vi "ExampleClient.vi"() -> ()   [LabVIEW 2017]
uses:
  Support/StreamClientState.ctl
  Controller/Support/StreamHeader.ctl
  jsonRPCwebservice/client/config.ctl
  Support/msg.ctl
  <userlib>/_SEH/Controls/CEH/CEH Actions.ctl
  Controller/Support/methods.ctl
  Support/globals.vi
  <vilib>/LVH/i3 JSON/JSON Parsing/Get Object Parameter Files/Get Object Parameter - Object.vi
  <vilib>/WebDAVClient/Simple Get File.vi
  jsonRPCwebservice/client/JSON_RPC_client.lvlib
  <vilib>/LVH/i3 JSON/i3-json.lvlib
  <vilib>/WebDAVClient/NI_WebDAV.lvlib
panel:
  in  "Trace":string
  in  "Tab Control":enum32{"Commands", "Stream", "Files"}(tab)
  in  "ToEcho":string
  in  "CheckConnection":bool
  in  "GoToSafeState":bool
  in  "GetResourceUsage":bool
  in  "echo":bool
  out "logging":bool
  out "Waveforms":sgl[][](graph)
  in  "Stream":bool
  in  "StreamAndLog":bool
  in  "StopStreaming":bool
  in  "ForceTigger":bool
  in  "RefreshLogFiles":bool
  in  "Logs":i32(listbox)
  in  "Download":bool
  in  "Exit":bool
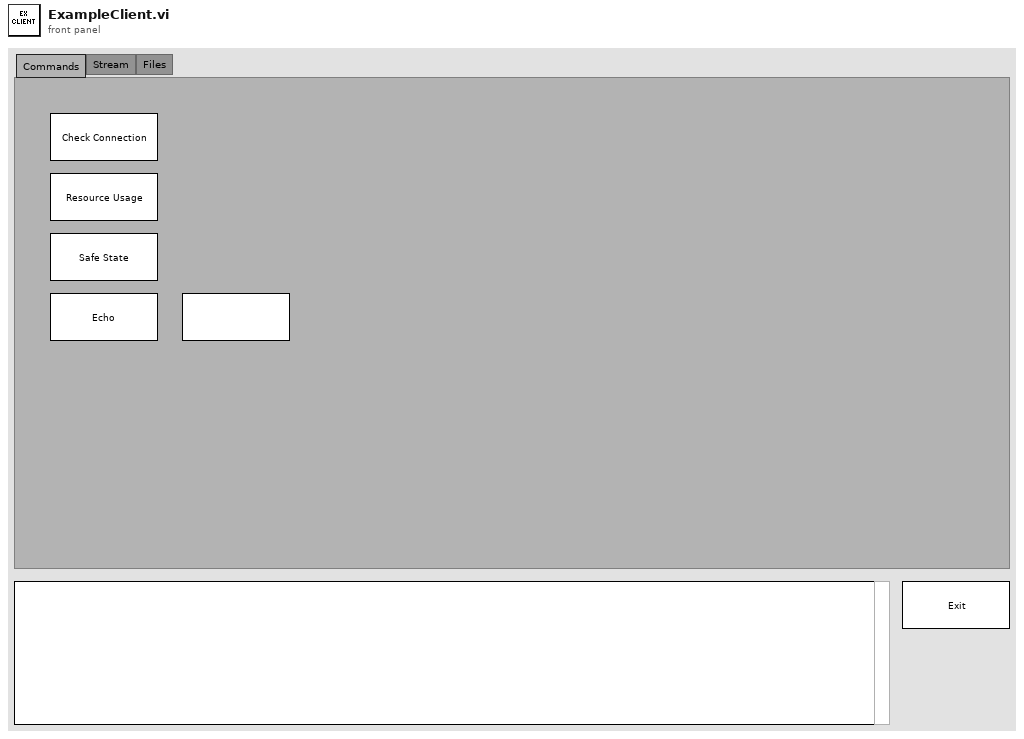
[diagram p1: front panel]
types:
  T1 = typedef "msg.ctl" = cluster{"cmd":string, "parameters":variant}
  T2 = typedef "JSON_RPC_client.lvlib/config.ctl" = cluster{"ip":string, "port":i32, "username":string, "password":string}
  T3 = typedef "StreamHeader.ctl" = cluster{"Channels":string[], "SampleRate":i32}
  T4 = typedef "StreamClientState.ctl" = enum16{"Initialize", "Idle", "ConnectAndOpen", "Connecting", "ReadHeader", "Streaming", "Disconnecting"}
  T5 = enum8{"Enabled", "Disabled", "Disabled and Grayed Out"}
  T6 = typedef "JSON_RPC_client.lvlib/reference.ctl" = cluster{"client handle":T7, "url":string}
  T7 = typedef "LabVIEWHTTPClient.lvlib/ClientHandle.ctl" = refnum<k1>
  T8 = enum16{"open", "open or create", "create or replace", "create", "open (read-only)"}
  T9 = typedef "methods.ctl" = enum16{"none", "echo", "GetResourceUsage", "CheckConnection", "GoToSafeState", "AvailableLogs", "ForceLogTrigger"}
  T10 = typedef "SEH Notification Info.ctl" = cluster{"Priority":i32, "Occurrences":i32, "First Occurrence":timestamp}
  T11 = typedef "CEH Actions.ctl" = enum16{"Log", "Display Error Message", "Safe State", "Shutdown"}
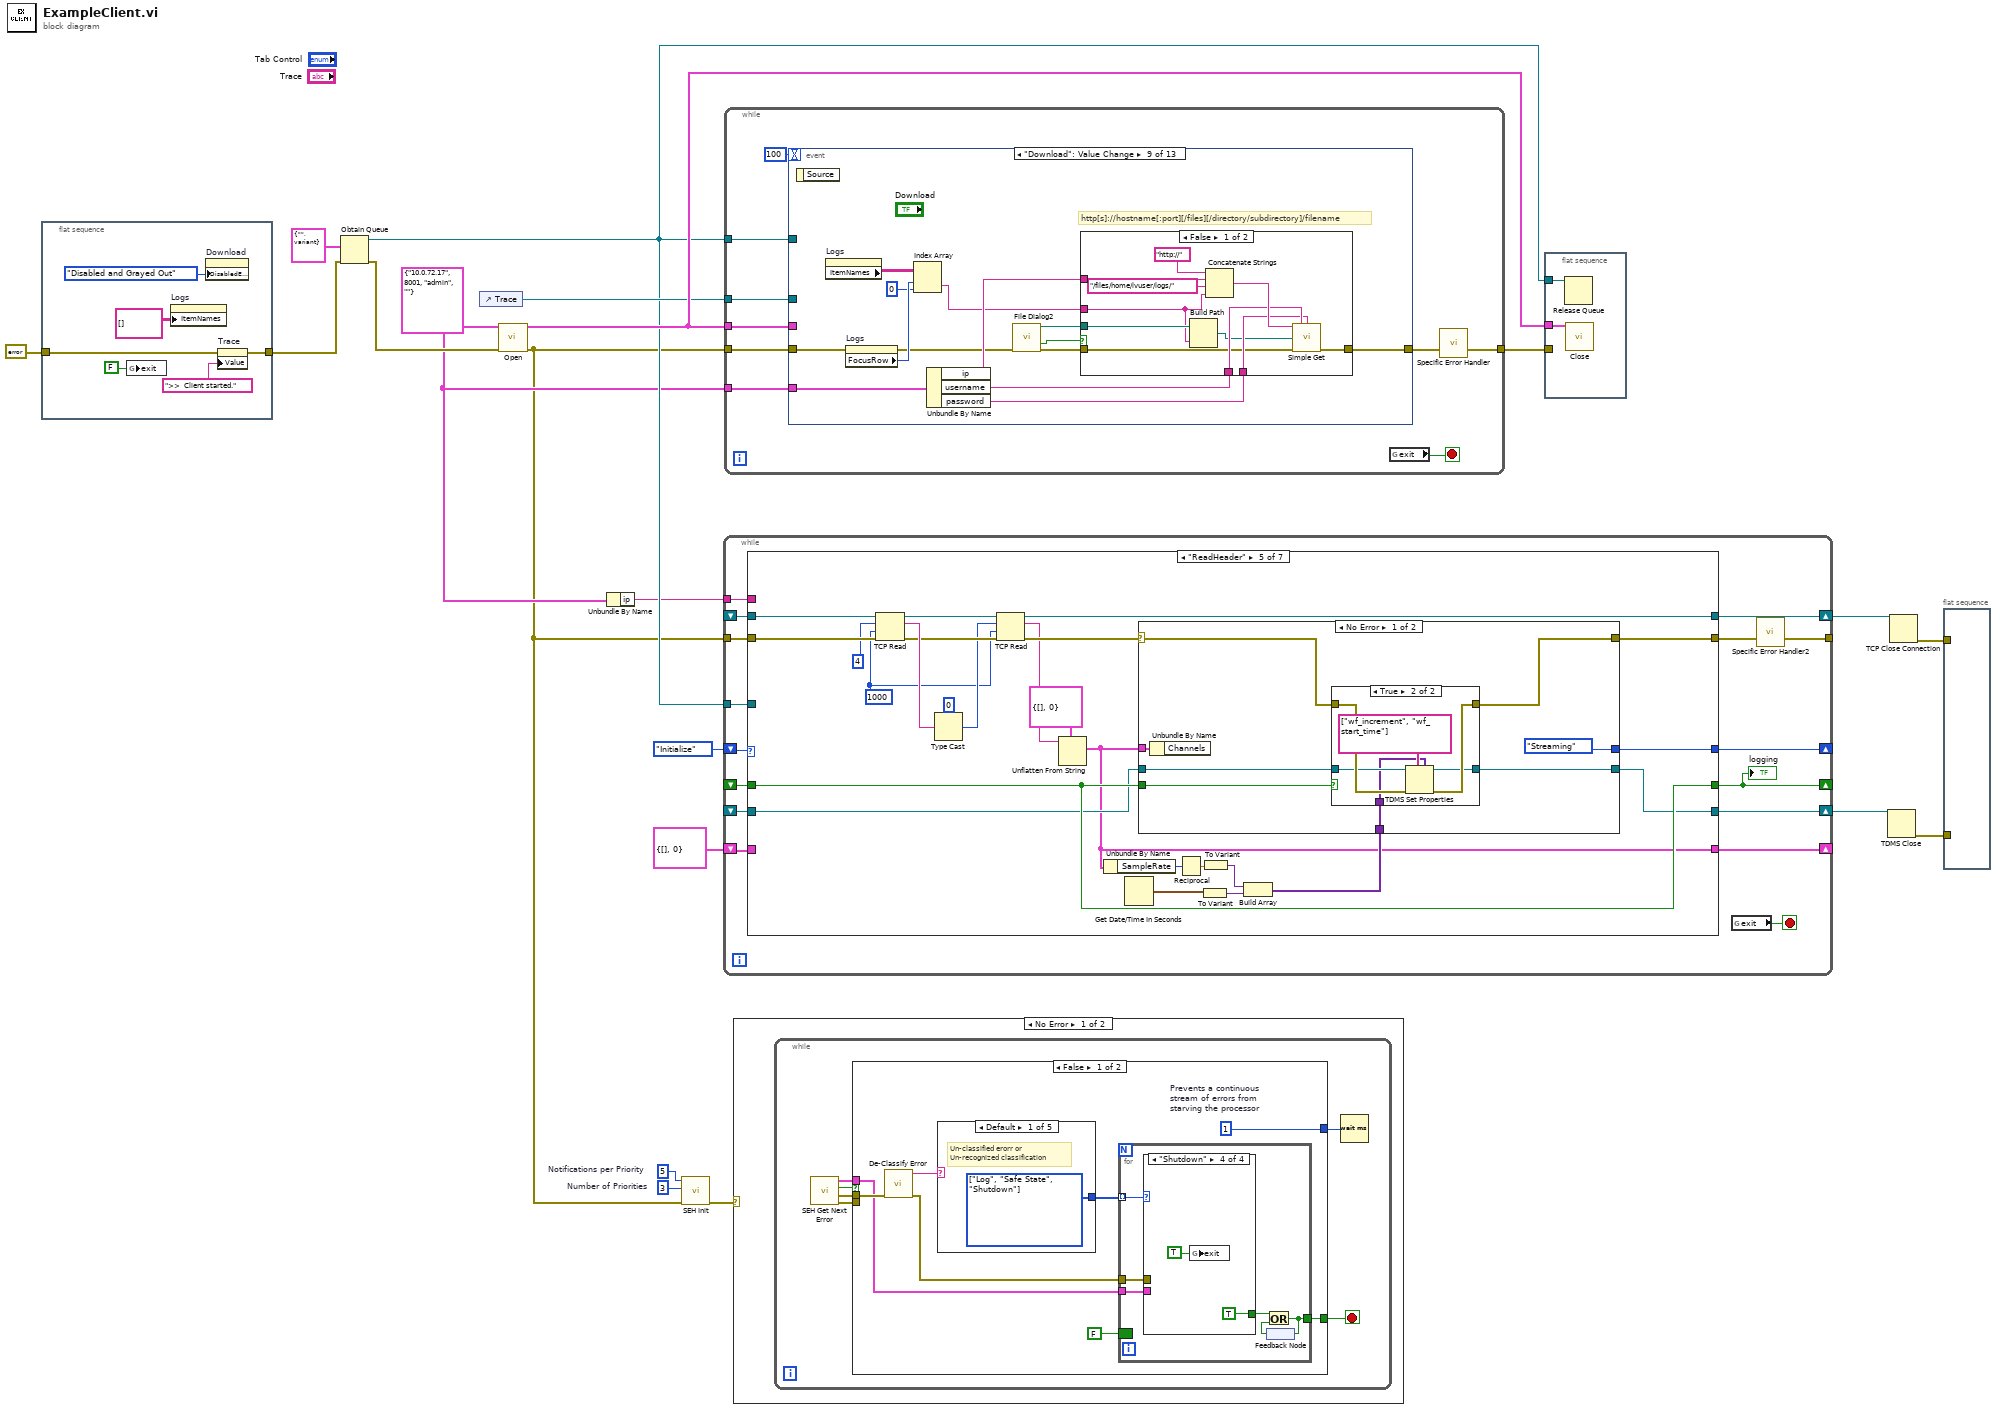
[diagram p0: block diagram]
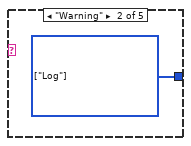
[diagram p2: hidden frame]
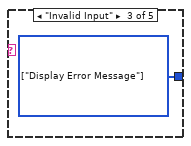
[diagram p3: hidden frame]
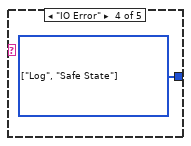
[diagram p4: hidden frame]
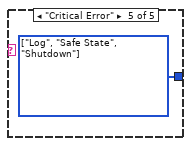
[diagram p5: hidden frame]
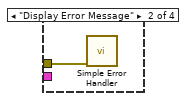
[diagram p7: hidden frame]
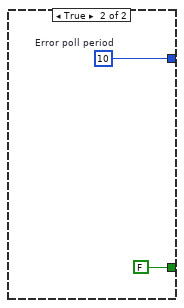
[diagram p9: hidden frame]
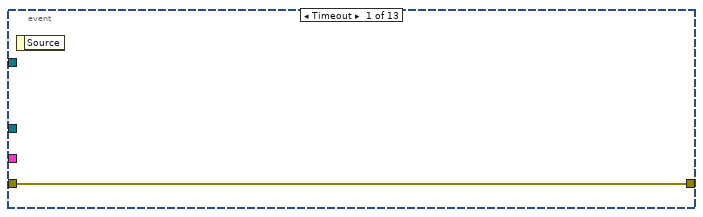
[diagram p11: hidden frame]
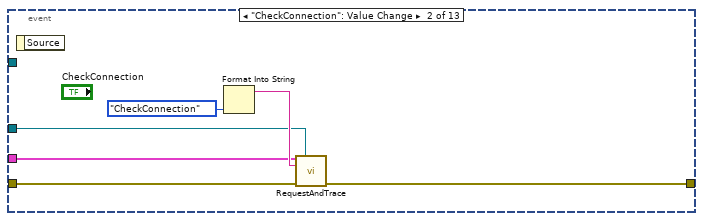
[diagram p12: hidden frame]
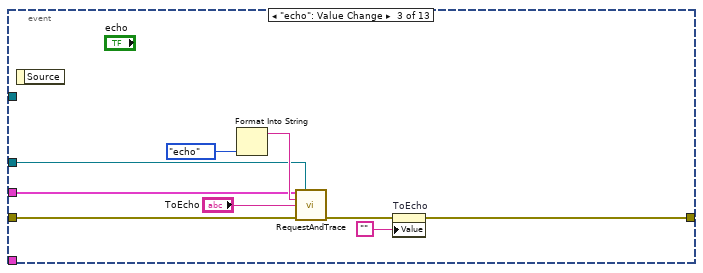
[diagram p13: hidden frame]
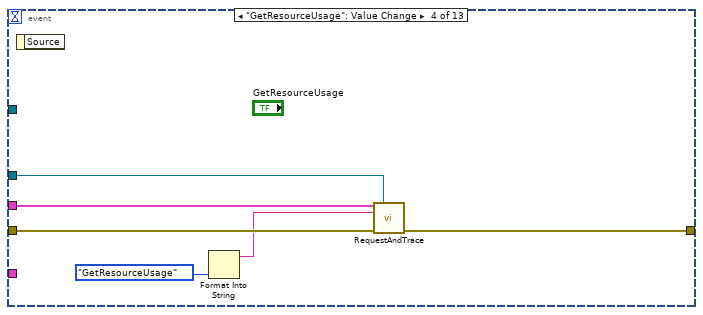
[diagram p14: hidden frame]
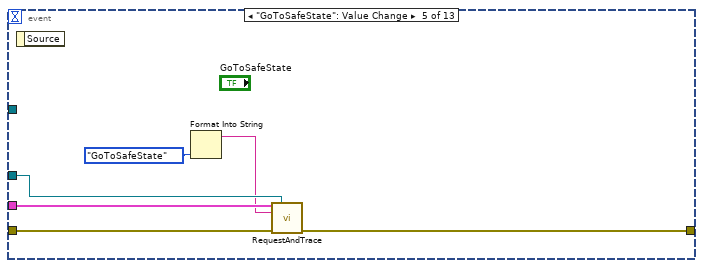
[diagram p15: hidden frame]
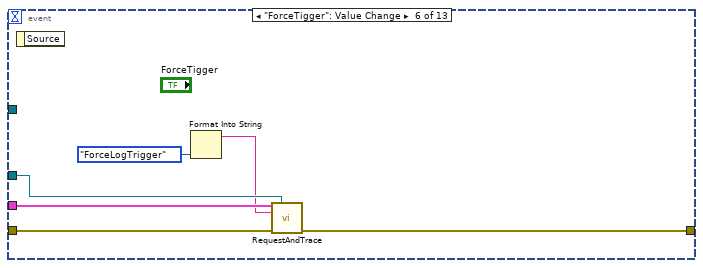
[diagram p16: hidden frame]
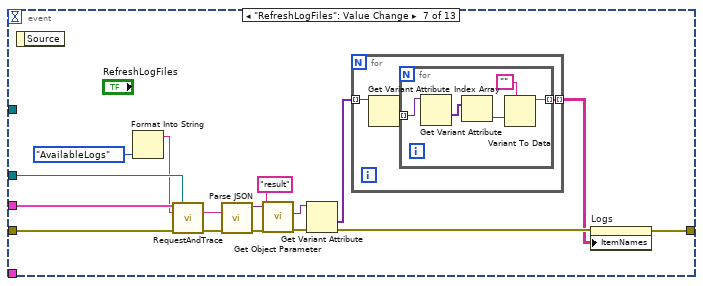
[diagram p17: hidden frame]
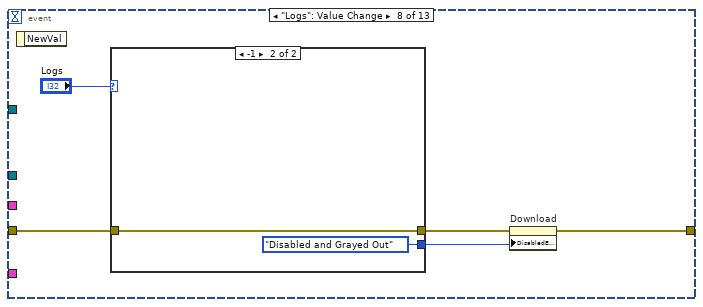
[diagram p18: hidden frame]
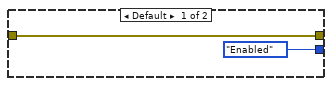
[diagram p19: hidden frame]
diagram:
  w8 = 3  # Number of Priorities
  w7 = 5  # Notifications per Priority
  w9 = T2 {"ip"="10.0.72.17", "port"=8001, "username"="admin", "password"=""} ("Connection")
  n1 = flat-sequence {
    tunnel: errorcluster {"status"=FALSE, "code"=0, "source"=""} ("error in (no error)") -> [w24]
    tunnel: [w23] -> w13
    frame #0 {
      n2 = global write "globals.vi" "exit"(FALSE ("exit")) -> ()
      n3 = property on="Logs" class="MCListbox (strict)"("ItemNames"=string[][] [] ("Item Names")) -> ()  [unwired: 2 in, 2 out]
      n4 = property on="Download" class="Bool"("DisabledEnum"=T5."Disabled and Grayed Out" ("Disabled")) -> ()  [unwired: 2 in, 2 out]
      n5 = property on="Trace" class="Str"(error in=w24, "Value"=">>  Client started." ("Trace")) -> (error out=w23:errorcluster)  [unwired: 1 in, 1 out]
    }
  }
  n6 = Obtain Queue(element data type=T1 {"cmd"="", "parameters"=variant} ("msg"), error in (no error)=w13) -> (queue out=w11:refnum<queue>, error out=w12:errorcluster)  [unwired: 3 in, 1 out]
  n7 = control-ref of="Trace"() -> (w15:refnum<vi>)
  n8 = call "Open.vi"("config"=w9, "error in (no error)"=w12) -> ("reference"=w18:T6, "error out"=w5:errorcluster)  [unwired: 12 in]
  n9 = Unbundle By Name(w9) -> ("ip"=w10:string)
  n10 = call <userlib>:"SEH Init.vi"("error in (no error)"=w5, "Number of Priorities"=w8, "Notifications per Priority"=w7) -> ("error out"=w6:errorcluster)  [unwired: 8 in]
  n11 = while {
    shift-right: [w41] -> _
    shift-left: StreamClientState."Initialize" ("StreamClientState") -> [w42]
    tunnel: w10 -> [w40]
    shift-right: [w38] -> w2
    shift-left: _ -> [w37]
    shift-right: [w36] -> _
    shift-left: T3 {"Channels"=[], "SampleRate"=0} ("StreamHeader") -> [w35]
    tunnel: w11 -> [w33]
    shift-right: [w27] -> _
    shift-left: _ -> [w32]
    shift-right: [w29] -> w1
    shift-left: _ -> [w28]
    tunnel: w5 -> [w39]
    tunnel: [w30] -> _
    stop <- w34 stop-if-true
    n12 = case shown="\"ReadHeader\"" w42 {
      tunnel: [StreamClientState."Idle" ("StreamClientState") w66 w109 w139 w161 w199 StreamClientState."Idle" ("StreamClientState")] -> w41
      tunnel: w40 -> [_ _ w108 w144 _ _ _]
      tunnel: w39 -> [w45 w62 w104 w138 w173 w220 _]
      tunnel: [w53 w57 w95 w130 w162 w200 w229] -> w31
      tunnel: [refnum<k5> refnum ("connection ID") refnum<k5> refnum ("connection ID") w106 w141 w164 w210 refnum<k5> refnum ("connection ID")] -> w38
      tunnel: w37 -> [_ _ _ _ w172 w219 w242]
      tunnel: [T3 {"Channels"=[], "SampleRate"=0} ("StreamHeader") T3 {"Channels"=[], "SampleRate"=0} ("StreamHeader") _ _ w149 w206 _] -> w36
      tunnel: w35 -> [_ _ _ _ _ w206 _]
      tunnel: w33 -> [_ w63 _ _ _ w198 _]
      tunnel: [FALSE w56 w107 w137 w153 w203 FALSE] -> w27
      tunnel: w32 -> [_ _ w107 w137 w153 w203 _]
      tunnel: [refnum<k34> refnum ("tdms file out") refnum<k34> refnum ("tdms file out") w100 refnum<k34> refnum ("tdms file out") w151 w202 refnum<k34> refnum ("tdms file out")] -> w29
      tunnel: w28 -> [_ _ _ _ w152 w202 w236]
      frame "Initialize" {
        n13 = property on="StreamAndLog" class="Bool"(error in=w45, "DisabledEnum"=T5."Enabled" ("Disabled")) -> (error out=w47:errorcluster)  [unwired: 1 in, 1 out]
        n14 = property on="Stream" class="Bool"(error in=w47, "DisabledEnum"=T5."Enabled" ("Disabled")) -> (error out=w49:errorcluster)  [unwired: 1 in, 1 out]
        n15 = property on="StopStreaming" class="Bool"(error in=w49, "DisabledEnum"=T5."Disabled and Grayed Out" ("Disabled")) -> (error out=w53:errorcluster)  [unwired: 1 in, 1 out]
      }
      frame "Idle", Default {
        n16 = Dequeue Element(queue=w63, timeout in ms (-1)=100, error in (no error)=w62) -> (element=w59:T1, timed out?=w60:bool, error out=w58:errorcluster)  [unwired: 1 out]
        n17 = case shown="True" w60 {
          tunnel: [w75 StreamClientState."Idle" ("StreamClientState")] -> w66
          tunnel: w59 -> [w74 _]
          tunnel: w58 -> [w72 w91]
          tunnel: [w69 w91] -> w57
          tunnel: [w67 FALSE] -> w56
          frame False {
            n18 = Unbundle By Name(w74) -> ("cmd"=w73:string)
            n19 = case shown="\"StartStream\"" w73 {
              selector: w73 -> [w80 _ _]
              tunnel: [StreamClientState."Idle" ("StreamClientState") StreamClientState."Connecting" ("StreamClientState") StreamClientState."ConnectAndOpen" ("StreamClientState")] -> w75
              tunnel: w72 -> [w77 w83 w88]
              tunnel: [w78 "Starting to stream" "Starting to log streaming data"] -> w70
              tunnel: [w77 w83 w88] -> w68
              tunnel: [FALSE FALSE TRUE] -> w67
              frame Default {
                n20 = Concatenate Strings(w80, " command ignored" ("string")) -> (w78:string)
              }
              frame "StartStream" {
              }
              frame "StartStreamAndLog" {
              }
            }
            n21 = control-ref of="Trace"() -> (w71:refnum<vi>)
            n22 = call "ToTrace.vi"("ToTrace"=w70, "TraceRef"=w71, "error in (no error)"=w68) -> ("error out"=w69:errorcluster)  [unwired: 12 in]
          }
          frame True {
          }
        }
      }
      frame "ConnectAndOpen" {
        w94 = T5."Disabled and Grayed Out" ("Disabled")
        w99 = "*.tdms" ("pattern label")
        n23 = call "File Dialog"("prompt"="Select a new stream fie location", "error in"=w104, "pattern (all files)"=w99, "pattern label"=w99) -> ("selected path"=w101:path, "cancelled"=w102:bool, "error out"=w103:errorcluster)  [unwired: 8 in, 1 out]
        n24 = case shown="False" w102 {
          tunnel: [w119 errorcluster {"status"=FALSE, "code"=0, "source"=""} ("error IO")] -> w98
          tunnel: [w118 StreamClientState."Disconnecting" ("StreamClientState")] -> w109
          tunnel: w108 -> [w117 _]
          tunnel: [w116 refnum<k5> refnum ("connection ID")] -> w106
          tunnel: w103 -> [w115 _]
          tunnel: w101 -> [w113 _]
          tunnel: [w110 _] -> w100
          frame False {
            n25 = TDMS Open(5:FALSE ("create index file? (T)"), 8:w115, 10:T8."create or replace" ("operation (0:open)"), 11:w113) -> (0:w114:errorcluster, 3:w110:refnum<k34>)  [unwired: 3 in]
            n26 = TCP Open Connection(address=w117, remote port or service name=u16 55550, timeout ms (60000)=5000, error in (no error)=w114) -> (connection ID=w116:refnum<k5>, error out=w120:errorcluster)  [unwired: 1 in]
            n27 = case shown="Error" w120 {
              selector: w120 -> [w124 w126]
              tunnel: [w124 w126] -> w119
              tunnel: [StreamClientState."ReadHeader" ("StreamClientState") StreamClientState."Disconnecting" ("StreamClientState")] -> w118
              frame No Error {
              }
              frame Error {
              }
            }
          }
          frame True {
          }
        }
        n28 = property on="Stream" class="Bool"(error in=w98, "DisabledEnum"=w94) -> (error out=w97:errorcluster)  [unwired: 1 in, 1 out]
        n29 = property on="StreamAndLog" class="Bool"(error in=w97, "DisabledEnum"=w94) -> (error out=w96:errorcluster)  [unwired: 1 in, 1 out]
        n30 = property on="StopStreaming" class="Bool"(error in=w96, "DisabledEnum"=T5."Enabled" ("Disabled")) -> (error out=w95:errorcluster)  [unwired: 1 in, 1 out]
      }
      frame "Connecting" {
        w133 = T5."Disabled and Grayed Out" ("Disabled")
        n31 = TCP Open Connection(address=w144, remote port or service name=u16 55550, timeout ms (60000)=5000, error in (no error)=w138) -> (connection ID=w141:refnum<k5>, error out=w140:errorcluster)  [unwired: 1 in]
        n32 = case shown="No Error" w140 {
          selector: w140 -> [w146 w148]
          tunnel: [w146 w148] -> w134
          tunnel: [StreamClientState."ReadHeader" ("StreamClientState") StreamClientState."Disconnecting" ("StreamClientState")] -> w139
          frame No Error {
          }
          frame Error {
          }
        }
        n33 = property on="Stream" class="Bool"(error in=w134, "DisabledEnum"=w133) -> (error out=w135:errorcluster)  [unwired: 1 in, 1 out]
        n34 = property on="StreamAndLog" class="Bool"(error in=w135, "DisabledEnum"=w133) -> (error out=w132:errorcluster)  [unwired: 1 in, 1 out]
        n35 = property on="StopStreaming" class="Bool"(error in=w132, "DisabledEnum"=T5."Enabled" ("Disabled")) -> (error out=w130:errorcluster)  [unwired: 1 in, 1 out]
      }
      frame "ReadHeader" {
        w165 = 1000 ("timeout ms (25000)")
        n36 = TCP Read(connection ID=w172, bytes to read=4, error in (no error)=w173, 9:w165) -> (connection ID out=w167:refnum<k5>, data out=w170:string, error out=w168:errorcluster)  [unwired: 1 in]
        n37 = Type Cast(type=0, x=w170) -> (*(type *) &x=w166:i32)
        n38 = TCP Read(connection ID=w167, bytes to read=w166, error in (no error)=w168, 9:w165) -> (connection ID out=w164:refnum<k5>, data out=w160:string, error out=w163:errorcluster)  [unwired: 1 in]
        n39 = Unflatten From String(type=T3 {"Channels"=[], "SampleRate"=0} ("StreamHeader"), binary string=w160) -> (value=w149:T3)  [unwired: 3 in, 2 out]
        n40 = Unbundle By Name(w149) -> ("SampleRate"=w150:i32)
        n41 = Get Date/Time In Seconds() -> (seconds since 1Jan1904=w157:timestamp)
        n42 = Reciprocal(x=w150) -> (1/x=w158:dbl)
        n43 = To Variant(anything=w157) -> (Variant=w155:variant)
        n44 = To Variant(anything=w158) -> (Variant=w156:variant)
        n45 = Build Array(w156, w155) -> (w154:variant[])
        n46 = case shown="No Error" w163 {
          selector: w163 -> [w180 w191]
          tunnel: [w179 w191] -> w162
          tunnel: [StreamClientState."Streaming" ("StreamClientState") StreamClientState."Disconnecting" ("StreamClientState")] -> w161
          tunnel: w152 -> [w178 w190]
          tunnel: [w177 w190] -> w151
          tunnel: w154 -> [w176 _]
          tunnel: w153 -> [w175 _]
          tunnel: w149 -> [w174 _]
          frame No Error {
            n47 = Unbundle By Name(w174) -> ()  [unwired: 1 out]
            n48 = case shown="True" w175 {
              tunnel: w180 -> [w182 w189]
              tunnel: [w182 w188] -> w179
              tunnel: w178 -> [w183 w187]
              tunnel: [w183 w186] -> w177
              tunnel: w176 -> [_ w184]
              frame False {
              }
              frame True {
                n49 = TDMS Set Properties(5:w184, 7:string[] ["wf_increment", "wf_start_time"] ("property names"), 8:w189, 11:w187) -> (0:w188:errorcluster, 3:w186:refnum<k34>)  [unwired: 2 in, 2 out]
              }
            }
          }
          frame Error {
          }
        }
      }
      frame "Streaming" {
        w212 = 1000 ("timeout ms (25000)")
        n50 = Dequeue Element(queue=w198, timeout in ms (-1)=0) -> (element=w195:T1, error out=w196:errorcluster)  [unwired: 1 in, 2 out]
        n51 = Unbundle By Name(w195) -> ("cmd"=w194:string)
        n52 = case shown="\"\"" w194 {
          tunnel: w196 -> [_ _ _]
          tunnel: [StreamClientState."Streaming" ("StreamClientState") StreamClientState."Streaming" ("StreamClientState") StreamClientState."Disconnecting" ("StreamClientState")] -> w193
          frame Default {
          }
          frame "" {
          }
          frame "StopStream" {
          }
        }
        n53 = TCP Read(connection ID=w219, bytes to read=4, error in (no error)=w220, 9:w212) -> (connection ID out=w214:refnum<k5>, data out=w217:string, error out=w215:errorcluster)  [unwired: 1 in]
        n54 = Type Cast(type=0, x=w217) -> (*(type *) &x=w213:i32)
        n55 = TCP Read(connection ID=w214, bytes to read=w213, error in (no error)=w215, 9:w212) -> (connection ID out=w210:refnum<k5>, data out=w211:string, error out=w207:errorcluster)  [unwired: 1 in]
        n56 = Type Cast(type=sgl[] [], x=w211) -> (*(type *) &x=w208:sgl[])
        n57 = call "FormatWaveforms.vi"("WaveformArray"=w208, "logFileRef"=w202, "log"=w203, "StreamHeader"=w206, "error in (no error)"=w207) -> ("Waveforms"=w204:sgl[][], "UpdateWaveforms"=w205:bool, "error out"=w201:errorcluster)  [unwired: 8 in]
        n58 = case shown="True" w205 {
          tunnel: w204 -> [_ w228]
          frame False {
          }
          frame True {
            "Waveforms" <- w228
          }
        }
        n59 = case shown="Error" w201 {
          selector: w201 -> [w225 w227]
          tunnel: [w225 w227] -> w200
          tunnel: [w224 StreamClientState."Disconnecting" ("StreamClientState")] -> w199
          tunnel: w193 -> [w224 _]
          frame No Error {
          }
          frame Error {
          }
        }
      }
      frame "Disconnecting" {
        w231 = T5."Enabled" ("Disabled")
        n60 = TDMS Close(11:w236) -> (0:w238:errorcluster)  [unwired: 1 in, 1 out]
        n61 = TCP Close Connection(connection ID=w242) -> (error out=w239:errorcluster)  [unwired: 2 in, 1 out]
        n62 = flat-sequence {
          tunnel: w239 -> [_]
          tunnel: w238 -> [_]
          frame #0 {
          }
        }
        n63 = property on="Stream" class="Bool"(error in=errorcluster {"status"=FALSE, "code"=0, "source"=""} ("error IO"), "DisabledEnum"=w231) -> (error out=w234:errorcluster)  [unwired: 1 in, 1 out]
        n64 = property on="StreamAndLog" class="Bool"(error in=w234, "DisabledEnum"=w231) -> (error out=w233:errorcluster)  [unwired: 1 in, 1 out]
        n65 = property on="StopStreaming" class="Bool"(error in=w233, "DisabledEnum"=T5."Disabled and Grayed Out" ("Disabled")) -> (error out=w229:errorcluster)  [unwired: 1 in, 1 out]
      }
    }
    "logging" <- w27
    n66 = global read "globals.vi" "exit"() -> (w34:bool)
    n67 = call "Specific Error Handler2"("Error to Check"=w31) -> ("error out"=w30:errorcluster)  [unwired: 11 in, 3 out]
  }
  n68 = while {
    tunnel: w18 -> [w251]
    tunnel: w15 -> [w245]
    tunnel: w11 -> [w244]
    tunnel: w9 -> [w243]
    tunnel: w5 -> [w250]
    tunnel: [w246] -> w16
    stop <- w248 stop-if-true
    n69 = event shown="[8] \"Download\": Value Change" {
      selector: _ -> [_ _ _ _ _ _ _ _ _ _ _ _ _]
      dyn-events: _ -> [_ _ _ _ _ _ _ _ _ _ _ _ _]
      timeout: 100 -> [_ _ _ _ _ _ _ _ _ _ _ _ _]
      tunnel: w251 -> [_ w254 w264 w272 w279 w285 w301 _ _ _ _ _ _]
      tunnel: w250 -> [w252 w257 w266 w271 w277 w283 w299 w312 w332 w347 w353 w360 _]
      tunnel: [w252 w256 w261 w268 w275 w281 w296 w313 w324 w346 w350 w356 errorcluster {"status"=TRUE, "code"=-1, "source"="User selected exit."} ("error out")] -> w247
      tunnel: w245 -> [_ w253 w263 w270 w276 w282 w298 _ _ _ w349 w358 _]
      tunnel: w244 -> [_ _ _ _ _ _ _ _ _ w348 w354 w361 _]
      tunnel: w243 -> [_ _ _ _ _ _ _ _ w328 _ _ _ _]
      event Timeout {
        n70 = event-data() -> ()  [unwired: 1 in, 1 out]
      }
      event "CheckConnection": Value Change {
        n71 = event-data() -> ()  [unwired: 1 in, 1 out]
        n72 = Format Into String(methods."CheckConnection" ("methods")) -> (resulting string=w255:string)  [unwired: 3 in, 1 out]
        n73 = call "RequestAndTrace.vi"("JSONRef in"=w254, "TraceRef"=w253, "method"=w255, "error in (no error)"=w257) -> ("error out"=w256:errorcluster)  [unwired: 9 in, 2 out]
      }
      event "echo": Value Change {
        n74 = event-data() -> ()  [unwired: 1 in, 1 out]
        n75 = Format Into String(methods."echo" ("methods")) -> (resulting string=w265:string)  [unwired: 3 in, 1 out]
        n76 = call "RequestAndTrace.vi"("JSONRef in"=w264, "TraceRef"=w263, "method"=w265, "params"="ToEcho", "error in (no error)"=w266) -> ("error out"=w262:errorcluster)  [unwired: 8 in, 2 out]
        n77 = property on="ToEcho" class="Str"(error in=w262, "Value"="") -> (error out=w261:errorcluster)  [unwired: 1 in, 1 out]
      }
      event "GetResourceUsage": Value Change {
        n78 = event-data() -> ()  [unwired: 1 in, 1 out]
        n79 = Format Into String(methods."GetResourceUsage" ("methods")) -> (resulting string=w269:string)  [unwired: 3 in, 1 out]
        n80 = call "RequestAndTrace.vi"("JSONRef in"=w272, "TraceRef"=w270, "method"=w269, "error in (no error)"=w271) -> ("error out"=w268:errorcluster)  [unwired: 9 in, 2 out]
      }
      event "GoToSafeState": Value Change {
        n81 = event-data() -> ()  [unwired: 1 in, 1 out]
        n82 = Format Into String(methods."GoToSafeState" ("methods")) -> (resulting string=w274:string)  [unwired: 3 in, 1 out]
        n83 = call "RequestAndTrace.vi"("JSONRef in"=w279, "TraceRef"=w276, "method"=w274, "error in (no error)"=w277) -> ("error out"=w275:errorcluster)  [unwired: 9 in, 2 out]
      }
      event "ForceTigger": Value Change {
        n84 = event-data() -> ()  [unwired: 1 in, 1 out]
        n85 = Format Into String(methods."ForceLogTrigger" ("methods")) -> (resulting string=w280:string)  [unwired: 3 in, 1 out]
        n86 = call "RequestAndTrace.vi"("JSONRef in"=w285, "TraceRef"=w282, "method"=w280, "error in (no error)"=w283) -> ("error out"=w281:errorcluster)  [unwired: 9 in, 2 out]
      }
      event "RefreshLogFiles": Value Change {
        n87 = event-data() -> ()  [unwired: 1 in, 1 out]
        n88 = Format Into String(methods."AvailableLogs" ("methods")) -> (resulting string=w297:string)  [unwired: 3 in, 1 out]
        n89 = call "RequestAndTrace.vi"("JSONRef in"=w301, "TraceRef"=w298, "method"=w297, "error in (no error)"=w299) -> ("reponse"=w294:string, "error out"=w295:errorcluster)  [unwired: 9 in, 1 out]
        n90 = call <vilib>:"Parse JSON.vi"("error in (no error)"=w295, "JSON String"=w294) -> ("error out"=w293:errorcluster, "JSON Tree"=w292:variant)  [unwired: 6 in, 2 out]
        n91 = call-poly <vilib>:"Get Object Parameter.vi"("error in (no error)"=w293, "Parameter Name"="result", "JSON Tree In (JSON Object)"=w292) -> ("error out"=w290:errorcluster, "JSON Object"=w289:variant)  [unwired: 5 in, 2 out]
        n92 = Get Variant Attribute(Variant=w289, error in=w290) -> (values=w287:variant[], error out=w288:errorcluster)  [unwired: 2 in, 2 out]
        n93 = for {
          tunnel: w287 -> [w302] mode=indexing
          tunnel: [w304] -> w286 mode=indexing
          n94 = Get Variant Attribute(Variant=w302) -> (values=w303:variant[])  [unwired: 3 in, 3 out]
          n95 = for {
            tunnel: [w308] -> w304 mode=indexing
            tunnel: w303 -> [w307] mode=indexing
            n96 = Get Variant Attribute(Variant=w307) -> (values=w306:variant[])  [unwired: 3 in, 3 out]
            n97 = Index Array(array=w306) -> (element=w305:variant)  [unwired: 1 in]
            n98 = Variant To Data(type="", Variant=w305) -> (data=w308:string)  [unwired: 1 in, 1 out]
          }
        }
        n99 = property on="Logs" class="MCListbox (strict)"(error in=w288, "ItemNames"=w286) -> (error out=w296:errorcluster)  [unwired: 1 in, 1 out]
      }
      event "Logs": Value Change {
        n100 = event-data() -> ()  [unwired: 1 in, 1 out]
        n101 = case shown="-1" "Logs" {
          tunnel: w312 -> [w316 w317]
          tunnel: [w316 w317] -> w311
          tunnel: [T5."Enabled" ("Disabled") T5."Disabled and Grayed Out" ("Disabled")] -> w310
          frame Default {
          }
          frame -1 {
          }
        }
        n102 = property on="Download" class="Bool"(error in=w311, "DisabledEnum"=w310) -> (error out=w313:errorcluster)  [unwired: 1 in, 1 out]
      }
      event "Download": Value Change {
        # "http[s]://hostname[:port][/files][/directory/subdirectory]/filename"
        n103 = event-data() -> ()  [unwired: 1 in, 1 out]
        n104 = property on="Logs" class="MCListbox (strict)"() -> ("ItemNames"=w330:string[][])  [unwired: 2 in, 2 out]
        n105 = property on="Logs" class="MCListbox (strict)"(error in=w332) -> (error out=w323:errorcluster, "FocusRow"=w331:i32)  [unwired: 1 in, 1 out]
        n106 = Index Array(array=w330, index (row)=w331, index (col)=0 ("index")) -> (element=w321:string)
        n107 = Unbundle By Name(w328) -> ("ip"=w327:string, "username"=w326:string, "password"=w325:string)
        n108 = call "File Dialog2"("error in"=w323) -> ("selected path"=w322:path, "cancelled"=w319:bool, "error out"=w320:errorcluster)  [unwired: 11 in, 1 out]
        n109 = case shown="False" w319 {
          tunnel: w327 -> [w342 _]
          tunnel: w326 -> [w339 _]
          tunnel: w325 -> [w338 _]
          tunnel: [w337 w344] -> w324
          tunnel: w322 -> [w336 _]
          tunnel: w321 -> [w335 _]
          tunnel: w320 -> [w333 w344]
          frame False {
            n110 = Build Path(base path=w336, name or relative path=w335) -> (appended path=w334:path)
            n111 = Concatenate Strings("http://" ("string"), w342, "/files/home/lvuser/logs/" ("string"), w335) -> (w340:string)
            n112 = call-poly <vilib>:"Simple Get.vi"("remote file uri"=w340, "username"=w339, "password"=w338, "local file path"=w334, "error in (no error)"=w333) -> ("error out"=w337:errorcluster)  [unwired: 9 in, 1 out]
          }
          frame True {
          }
        }
      }
      event "Stream": Value Change {
        n113 = event-data() -> ()  [unwired: 1 in, 1 out]
        n114 = Enqueue Element(queue=w348, element=T1 {"cmd"="StartStream", "parameters"=variant}, error in (no error)=w347) -> (error out=w346:errorcluster)  [unwired: 1 in, 2 out]
      }
      event "StreamAndLog": Value Change {
        n115 = event-data() -> ()  [unwired: 1 in, 1 out]
        n116 = Enqueue Element(queue=w354, element=T1 {"cmd"="StartStreamAndLog", "parameters"=variant}, error in (no error)=w353) -> (error out=w351:errorcluster)  [unwired: 1 in, 2 out]
        n117 = call "ToTrace.vi"("ToTrace"="Stream and log started.", "TraceRef"=w349, "error in (no error)"=w351) -> ("error out"=w350:errorcluster)  [unwired: 12 in]
      }
      event "StopStreaming": Value Change {
        n118 = event-data() -> ()  [unwired: 1 in, 1 out]
        n119 = Enqueue Element(queue=w361, element=T1 {"cmd"="StopStream", "parameters"=variant}, error in (no error)=w360) -> (error out=w359:errorcluster)  [unwired: 1 in, 2 out]
        n120 = call "ToTrace.vi"("ToTrace"="Streaming stopped.", "TraceRef"=w358, "error in (no error)"=w359) -> ("error out"=w356:errorcluster)  [unwired: 12 in]
      }
      event "Exit": Value Change {
        n121 = event-data() -> ()  [unwired: 1 in, 1 out]
      }
    }
    n122 = global read "globals.vi" "exit"() -> (w248:bool)
    n123 = call "Specific Error Handler"("Error to Check"=w247) -> ("error out"=w246:errorcluster)  [unwired: 11 in, 3 out]
  }
  n124 = case shown="No Error" w6 {
    frame No Error {
      n125 = while {
        stop <- w368 stop-if-true
        n126 = call <userlib>:"SEH Get Next Error.vi"() -> ("Transmission Error"=w364:errorcluster, "Transmitted Error"=w367:errorcluster, "Empty?"=w366:bool, "Notification Info"=w365:T10)  [unwired: 8 in]
        n127 = case shown="False" w366 {
          tunnel: [w377 w393] -> w369
          tunnel: w367 -> [w376 _]
          tunnel: w365 -> [w372 _]
          tunnel: [w371 FALSE] -> w368
          tunnel: w364 -> [_ _]
          frame False {
            w377 = u32 1  # Prevents a continuous stream of errors from starving the processor
            n128 = call <userlib>:"De-Classify Error.vi"("Classified Error"=w376) -> ("De-Classified Error"=w374:errorcluster, "Error Classification"=w375:string)  [unwired: 8 in, 1 out]
            n129 = case shown="Default" w375 {
              tunnel: [w378 w379 w380 w381 w382] -> w373
              frame Default {
                w378 = T11[] [enum."Log", enum."Safe State", enum."Shutdown"] items=["Log", "Display Error Message", "Safe State", "Shutdown"]
                # "Un-classified erorr or\nUn-recognized classification"
              }
              frame "Warning" {
                w379 = T11[] [enum."Log"] items=["Log", "Display Error Message", "Safe State", "Shutdown"]
              }
              frame "Invalid Input" {
                w380 = T11[] [enum."Display Error Message"] items=["Log", "Display Error Message", "Safe State", "Shutdown"]
              }
              frame "IO Error" {
                w381 = T11[] [enum."Log", enum."Safe State"] items=["Log", "Display Error Message", "Safe State", "Shutdown"]
              }
              frame "Critical Error" {
                w382 = T11[] [enum."Log", enum."Safe State", enum."Shutdown"] items=["Log", "Display Error Message", "Safe State", "Shutdown"]
              }
            }
            n130 = for {
              tunnel: w374 -> [w387]
              tunnel: w373 -> [w388] mode=indexing
              tunnel: w372 -> [w386]
              border: FALSE -> [_]
              tunnel: [w383] -> w371
              n131 = case shown="\"Shutdown\"" w388 {
                tunnel: w387 -> [_ w389 _ _]
                tunnel: w386 -> [_ _ _ _]
                tunnel: [_ _ _ TRUE] -> w385
                frame "Log", Default {
                  # "Implement log \nhere"
                }
                frame "Display Error Message" {
                  n132 = call <vilib>:"Simple Error Handler.vi"("error in (no error)"=w389) -> ()  [unwired: 4 in, 5 out]
                }
                frame "Safe State" {
                  # "Implement safe\nstate here"
                }
                frame "Shutdown" {
                  n133 = global write "globals.vi" "exit"(TRUE ("exit")) -> ()
                }
              }
              n134 = feedback #1() -> (w384:bool)
              n135 = Or(x=w385, y=w384) -> (x .or. y?=w383:bool)
              n136 = feedback-in #1(w383) -> ()
            }
          }
          frame True {
            w393 = u32 10  # Error poll period
          }
        }
        n137 = Wait (ms)(milliseconds to wait=w369) -> ()  [unwired: 1 out]
      }
    }
    frame Error {
      # "Error notification cannot initialize\n(log this)"
    }
  }
  n138 = flat-sequence {
    tunnel: w18 -> [w395]
    tunnel: w16 -> [_]
    tunnel: w11 -> [w394]
    frame #0 {
      n139 = Release Queue(queue=w394) -> ()  [unwired: 2 in, 3 out]
      n140 = call "Close.vi"("reference in"=w395) -> ()  [unwired: 14 in, 1 out]
    }
  }
  n141 = TDMS Close(11:w1) -> (0:w3:errorcluster)  [unwired: 1 in, 1 out]
  n142 = TCP Close Connection(connection ID=w2) -> (error out=w4:errorcluster)  [unwired: 2 in, 1 out]
  n143 = flat-sequence {
    tunnel: w4 -> [_]
    tunnel: w3 -> [_]
    frame #0 {
    }
  }
